vi "Stepper.vi"(8 "error in (no error)":errorcluster) -> (0 "error out":errorcluster, 3 "Stepper out":refnum<class "Stepper.lvclass">)   [LabVIEW 2017, in "Stepper.lvclass"]
uses:
  Stepper.lvclass
  Stepper.lvclass/Stepper.ctl
  <vilib>/Utility/config.llb/Read Key (Double).vi
  <vilib>/DAQmx/create/channels.llb/DAQmx Create Channel (DO-Digital Output).vi
  <vilib>/Utility/config.llb/NI_LVConfig.lvlib
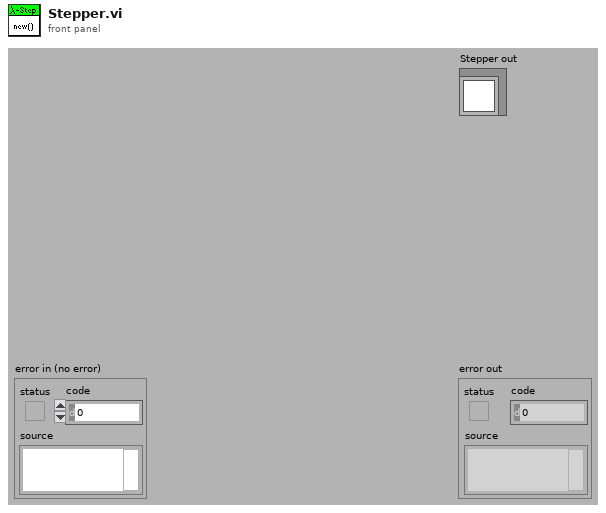
[diagram p1: front panel]
types:
  T1 = typedef "NI_LVConfig.lvlib/Config Data RefNum.ctl" = refnum<k1>
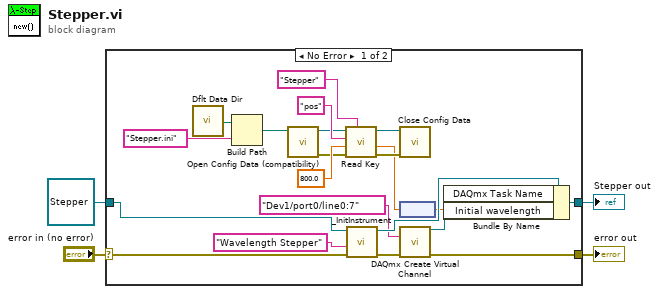
[diagram p0: block diagram]
diagram:
  n1 = case shown="No Error" "error in (no error)" {
    selector: "error in (no error)" -> [w24 w27]
    tunnel: [w19 w27] -> w3
    tunnel: [w18 w26] -> w1
    tunnel: refnum<class "Stepper.lvclass"> refnum ("Stepper in") -> [w25 w26]
    frame No Error {
      n2 = call <vilib>:"Dflt Data Dir.vi"() -> ("App:Default Data Directory"=w8:path)
      n3 = Build Path(base path=w8, name or relative path="Stepper.ini") -> (appended path=w10:path)
      n4 = call <vilib>:"Open Config Data (compatibility).vi"("configuration file path"=w10) -> ("error out"=w12:errorcluster, "refnum"=w11:T1)  [unwired: 8 in, 1 out]
      n5 = call-poly <vilib>:"Read Key.vi"("section"="Stepper", "error in (no error)"=w12, "default value"=800.0, "key"="pos", "refnum"=w11) -> ("error out"=w15:errorcluster, "value"=w7:dbl, "refnum out"=w14:T1)  [unwired: 4 out]
      n6 = call-dynamic "_InitInstrument.vi"("error in (no error)"=w24, "Name"="Wavelength Stepper", "Instrument in"=w25) -> ("error out"=w20:errorcluster, "Instrument out"=w23:refnum<class "Stepper.lvclass">)  [unwired: 3 in, 4 out]
      n7 = call <vilib>:"Close Config Data.vi"("error in (no error)"=w15, "refnum"=w14) -> ()  [unwired: 1 in, 9 out]
      n8 = node(w7) -> (w6:dbl[unit])
      n9 = call-poly <vilib>:"DAQmx Create Virtual Channel.vi"("lines"=tag "Dev1/port0/line0:7" ("task in"), "error in"=w20) -> ("task out"=w17:refnum<k21>, "error out"=w19:errorcluster)  [unwired: 4 in, 8 out]
      n10 = Bundle By Name(cluster=w23, "DAQmx Task Name"=w17, "Initial wavelength"=w6) -> (w18:refnum<class "Stepper.lvclass">)
    }
    frame Error {
    }
  }
  "error out" <- w3
  "Stepper out" <- w1
